vi "Remove Duplicate Consecutive Vertices.vi"(8 "Error In":errorcluster, 11 "Freehand Line Points (in)":i32[](array[numeric])) -> (0 "Error Out":errorcluster, 3 "Freehand Line Points (out)":i32[](array[numeric]))   [LabVIEW 2021, in "Image.lvlib"]
uses:
  Image.lvlib
panel:
  out "# Duplicates":i32
  out "# Vertices":i32
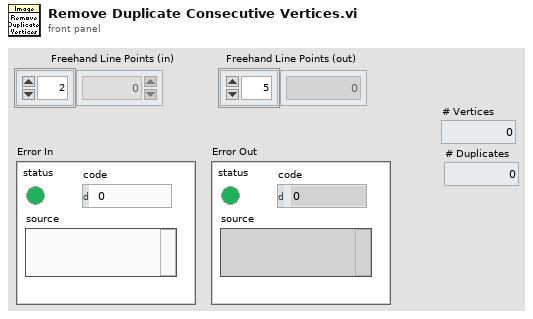
[diagram p1: front panel]
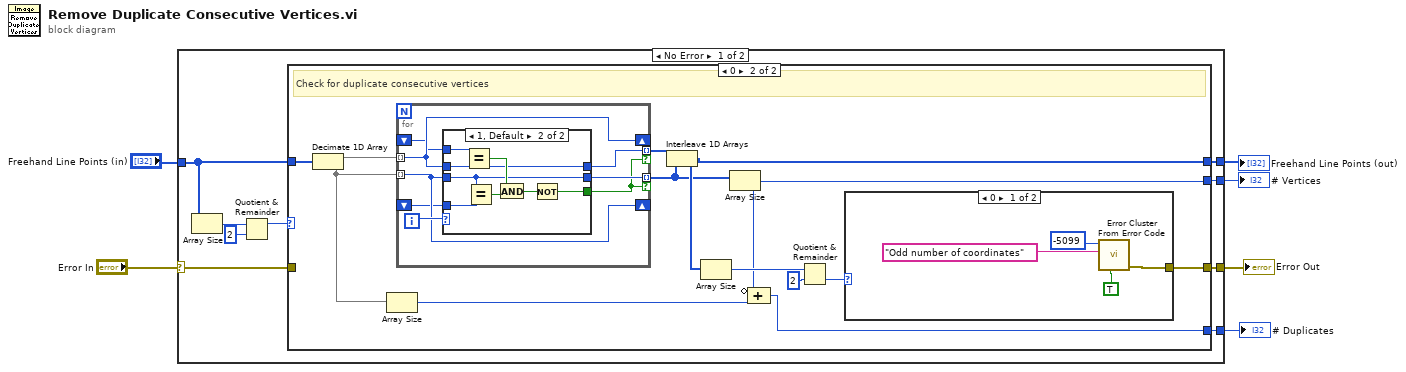
[diagram p0: block diagram]
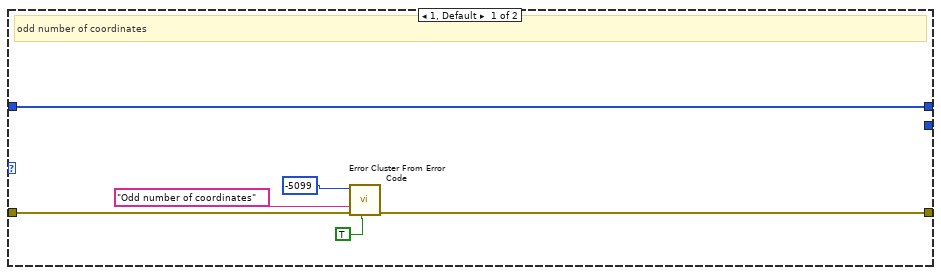
[diagram p2: hidden frame]
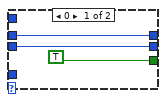
[diagram p4: hidden frame]
diagram:
  n1 = case shown="No Error" "Error In" {
    selector: "Error In" -> [w10 w59]
    tunnel: "Freehand Line Points (in)" -> [w15 w58]
    tunnel: [w11 w58] -> w5
    tunnel: [w9 w59] -> w3
    tunnel: [w8 _] -> w2
    tunnel: [w7 _] -> w1
    frame No Error {
      n2 = Array Size(array=w15) -> (size(s)=w14:i32)
      n3 = Quotient & Remainder(x=w14, y=2) -> (x-y*floor(x/y)=w12:i32)  [unwired: 1 out]
      n4 = case shown="0" w12 {
        tunnel: w15 -> [w21 w34]
        tunnel: [w21 w31] -> w11
        tunnel: w10 -> [w20 _]
        tunnel: [w19 w28] -> w9
        tunnel: [_ w22] -> w8
        tunnel: [_ w24] -> w7
        frame 1, Default {
          # "odd number of coordinates"
          n5 = call <vilib>:"Error Cluster From Error Code.vi"("show call chain? (False)"=TRUE, "error in (no error)"=w20, "error message (\"\")"="Odd number of coordinates" ("error message (\"\")"), "error code (0)"=-5099) -> ("error out"=w19:errorcluster)  [unwired: 5 in]
        }
        frame 0 {
          # "Check for duplicate consecutive vertices"
          n6 = Decimate 1D Array(w34) -> (w33:i32[], w27:i32[])
          n7 = Array Size(array=w27) -> (size(s)=w26:i32)
          n8 = for {
            tunnel: w33 -> [w45] mode=indexing
            tunnel: w27 -> [w43] mode=indexing
            shift-right: [w45] -> _
            shift-left: _ -> [w40]
            shift-right: [w43] -> _
            shift-left: _ -> [w39]
            tunnel: [w44] -> w32 mode=indexing if=w41
            tunnel: [w42] -> w23 mode=indexing if=w41
            i -> [w46]
            n9 = case shown="1, Default" w46 {
              tunnel: w45 -> [w49 w51]
              tunnel: [w49 w51] -> w44
              tunnel: w43 -> [w48 w50]
              tunnel: [w48 w50] -> w42
              tunnel: [TRUE w52] -> w41
              tunnel: w40 -> [_ w57]
              tunnel: w39 -> [_ w56]
              frame 0 {
              }
              frame 1, Default {
                n10 = Equal?(x=w57, y=w51) -> (x = y?=w55:bool)
                n11 = Equal?(x=w50, y=w56) -> (x = y?=w54:bool)
                n12 = And(x=w55, y=w54) -> (x .and. y?=w53:bool)
                n13 = Not(x=w53) -> (.not. x?=w52:bool)
              }
            }
          }
          n14 = Interleave 1D Arrays(w32, w23) -> (w31:i32[])
          n15 = Array Size(array=w31) -> (size(s)=w25:i32)
          n16 = Array Size(array=w23) -> (size(s)=w22:i32)
          n17 = Compound Arithmetic op=ADD(invert w22, w26) -> (w24:i32)
          n18 = Quotient & Remainder(x=w25, y=2) -> (floor(x/y)=w29:i32)  [unwired: 1 out]
          n19 = case shown="0" w29 {
            tunnel: [w36 _] -> w28
            frame 0 {
              n20 = call <vilib>:"Error Cluster From Error Code.vi"("show call chain? (False)"=TRUE, "error message (\"\")"="Odd number of coordinates" ("error message (\"\")"), "error code (0)"=-5099) -> ("error out"=w36:errorcluster)  [unwired: 6 in]
            }
            frame 1, Default {
            }
          }
        }
      }
    }
    frame Error {
    }
  }
  "Freehand Line Points (out)" <- w5
  "Error Out" <- w3
  "# Vertices" <- w2
  "# Duplicates" <- w1
